vi "Current_and_Spectrum_View.vi"() -> ()   [LabVIEW 2009]
doc: "I. Description:\nThis example demonstrates how to perform an analog software triggered acquisition. The example allows the user to specify the triggering condition and the number of pre-trigger samples to acquire.\n \nII. Instructions for Running:\n1. Select the physical channel to correspond to where your signal is input on the DAQ device.\n2. Enter the minimum and maximum voltage ranges.\nNote: For better accuracy try to match the Input Ranges to the expected voltage level of the measured signal.\n3. Specify the rate of the sample clock. \n4. Specify the number of samples to read per iteration of the continuous input operation. These samples will then be monitored for the trigger condition. The trigger condition is determined by the parameters explained below.\n5. Specify the index of the channel that will be monitored for the requested condition. The first channel in the scan list will have an index equals to 0. It's possible to verify the name of the selected channel once the VI is run, after setting the Channel Index value.\n6. Set the triggering condition to be applied to the channel specified by the Channel Index value. The conditions created for this example are:\n\n- Rising Edge: The trigger condition is met as soon as the monitored signal falls below the Hysteresis window and then crosses past the specified Level.\n- Falling Edge: The trigger condition is met as soon as the monitored signal rises above the Hysteresis window and then crosses past the specified Level.\n- Above Level: The trigger condition is met as soon as the monitored signal is above the specified Level. \n- Below Level: The trigger condition is met as soon as the monitored signal is below the specified Level.\n- When Inside Window: The trigger condition is met as soon as the monitored signal is within the specified window.\n- When Outside Window: The trigger condition is met as soon as the monitored signal is not within the specified window.\n\n7. Set the Level value to be used by the selected condition.\n8. Set the Window Amplitude/ Hysteresis to be used by the Window/Edge conditions\n\n- The upper limit of the conditional window is calculated by adding the Window Amplitude to the condition Level.\n- The lower limit of the conditional window is calculated by subtracting the Window Amplitude from the condition Level.\n- The Hysteresis window for the Rising Edge condition is defined as Level minus the Hysteresis value. \n- The Hysteresis window for the Falling Edge condition is defined as Level plus the Hysteresis value.\n\n8. Set the number of pre-trigger samples if desired.\n\nIII. Block Diagram Steps:\n1. Create an analog input voltage channel.\n2. Find out how many channels are being used in this operation.\n3. Define the Sample Clock Rate. Additionally, define the sample mode to be continuous.\n4. Show the Channel Name of the Condition Channel.\n5. Initialize the data arrays to be used for holding successive iterations of data. This pre-allocation of memory improves the performance of the application. Refer to the VI documentation for more information.\n\nNOTE: The number of samples that meet the triggering condition is not fixed; it depends on the value of the monitored signal. This means that the number of samples to be returned by Analog Trigger Through Software (Scaled).VI may vary from one iteration to the next. In order to avoid dynamically allocating memory while filtering the data (a process that creates), this example pre-allocates arrays for the data before the acquisition starts. The arrays are initialized to the maximum number of elements expected per iteration.\n\n6. Call the Start VI to start the acquisition.\n7. Read the scaled analog input data.\nNote: The Shift Registers attached to the While Loop are used to keep track of triggering status and previous data samples (needed for pre-triggered acquisitions). \n8. Use the Analog Trigger Through Software (Scaled).VI specifically created for this example to detect the requested trigger condition through software.\n9. Show the acquired data if the trigger condition is met.\n10. Stop the loop if the trigger condition is met, an error occurs or the Stop button is pressed. \n11. Call the Clear Task VI to clear the Task.\n12. Use the popup dialog box to display an error or warning if any.\n\nIV. I/O Connections Overview:\nMake sure your signal input terminal matches the Physical Channel I/O control. For further connection information, refer to your hardware reference manual."
uses:
  <vilib>/Utility/error.llb/DialogType.ctl
  <vilib>/DAQmx/configure/timing.llb/DAQmx Timing (Sample Clock).vi
  <vilib>/DAQmx/create/channels.llb/DAQmx Create Channel (AI-Voltage-Basic).vi
  <vilib>/DAQmx/read.llb/DAQmx Read (Analog 2D DBL NChan NSamp).vi
  <vilib>/express/express analysis/Spectral/XNode/ExpressSpectralMeasurementsBlockNode.xnode
  <vilib>/express/express analysis/Spectral/Block/exnSpectralBlock spectral measurements power poly.vi
  <vilib>/express/express analysis/Spectral/Block/exnSpectralBlock spectral measurements power DDT.vi
panel:
  out "x/y":dbl[](array[numeric])
  out "Waveform Graph 2":dynamicdata(graph)
  out "# Pretrigger Samples\nAcquired":i32
  out "Waveform Graph":dbl[][](graph)
  out "Pre-Trigger Error Indicator":bool caption="Error Indicator\n(Indicates if trigger occurs before\npre-trigger samples were acquired)"
  in  "Pretrigger Samples":i32
  in  "Window Amplitude":dbl=0.5 caption="Window Amplitude\n/Hysteresis" step=0.10000000149011612 format="%.2p"
  out "Channel Name":string
  in  "Condition":T1(ring)=enum."Above Level"
  in  "Channel Index":i32
  in  "Level":dbl=-11.0 step=0.10000000149011612 format="%.2p"
  in  "Samples to Read":i32=40000 caption="Samples to Read per Iteration"
  in  "Maximum Value":dbl=10.0 format="%.2p"
  in  "Minimum Value":dbl=-10.0 format="%.2p"
  in  "Physical Channel":tag="Dev1/ai0"
  in  "Rate":dbl=10000.0 caption="Sample Rate (Hz)" format="%0.2f"
  in  "Stop":bool caption="stop"
  # "For instructions, select Help>>Show Context Help"
  # "Channel Parameters"
  # "Timing Parameters"
  # "Triggering Parameters"
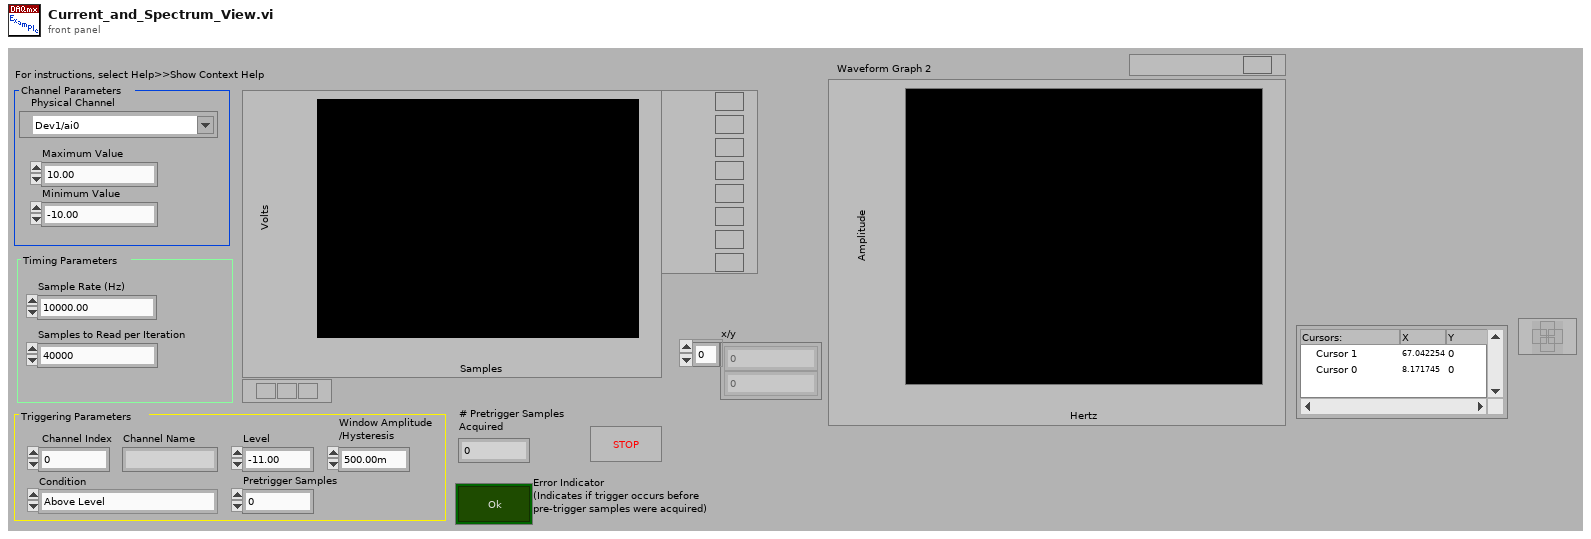
[diagram p1: front panel]
types:
  T1 = enum16{"Rising Edge", "Falling Edge", "Above Level", "Below Level", "When Inside Window", "When Outside Window"}
  T2 = typedef "DialogType.ctl" = u16
  T3 = cluster{"averaging mode":u16, "weighting mode":u16, "number of averages":u32}
  T4 = cluster{"dB On (F)":bool, "unwrap phase (F)":bool, "convert to degree (F)":bool}
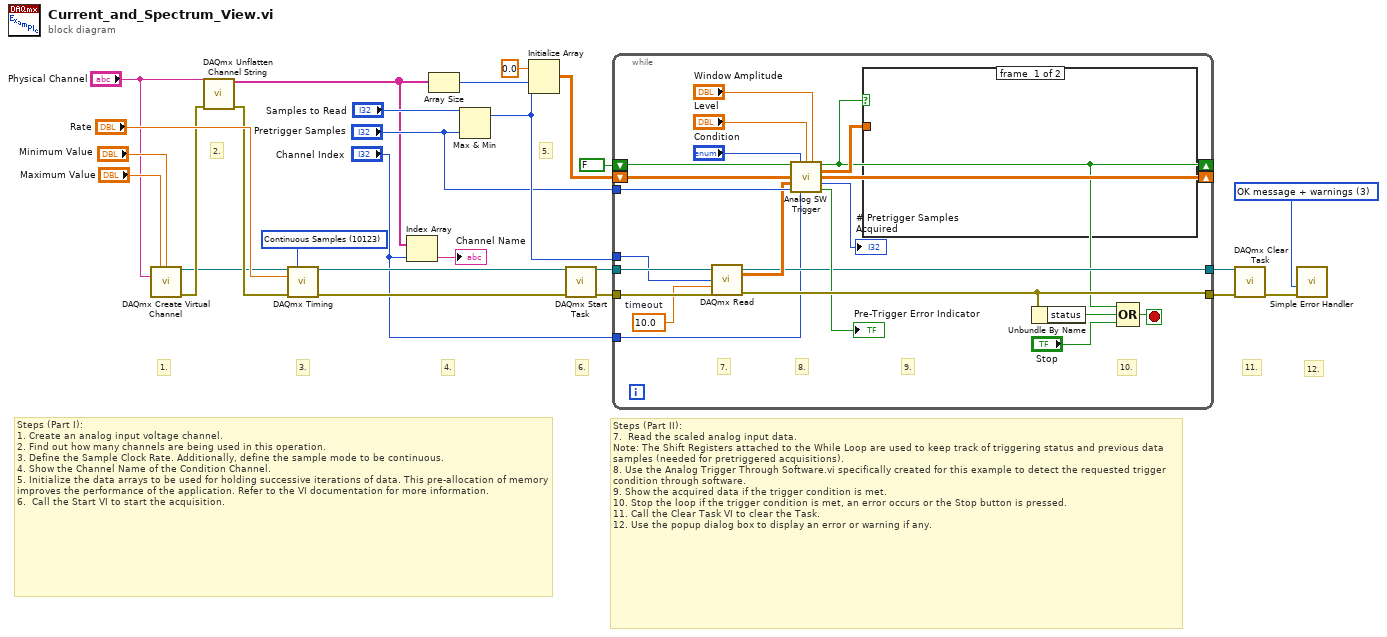
[diagram p0: block diagram]
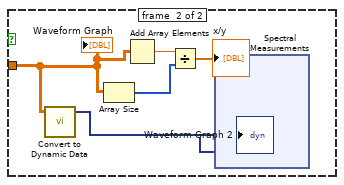
[diagram p2: hidden frame]
diagram:
  w20 = T2 3 items=["no dialog", "OK message", "continue or stop message", "OK message + warnings", "continue/stop + warnings"] ("type of dialog (OK msg:1)")
  w21 = 10123 items=["Finite Samples"=10178, "Continuous Samples"=10123] ("sample mode")
  # "5."
  # "3."
  # "Steps (Part II): \n7.  Read the scaled analog input data.\nNote: The Shift Registers attached to the While Loop are used to keep track of triggering status and previous data samples (needed for pretriggered acquisitions). \n8. Use the Analog Trigger Through Software.vi specifically created for this example to detect the requested trigger condition through software.\n9. Show the acquired data if the trigger condition is met.\n10. Stop the loop if the trigger condition is met, an error occurs or the Stop button is pressed. \n11. Call the Clear Task VI to clear the Task.\n12. Use the popup dialog box to display an error or warning if any."
  # "4."
  # "12."
  # "Steps (Part I): \n1. Create an analog input voltage channel.\n2. Find out how many channels are being used in this operation.\n3. Define the Sample Clock Rate. Additionally, define the sample mode to be continuous.\n4. Show the Channel Name of the Condition Channel.\n5. Initialize the data arrays to be used for holding successive iterations of data. This pre-allocation of memory improves the performance of the application. Refer to the VI documentation for more information.\n6.  Call the Start VI to start the acquisition."
  # "11."
  # "6."
  # "2."
  # "1."
  n1 = call-poly <vilib>:"DAQmx Create Virtual Channel.vi"("maximum value"="Maximum Value", "minimum value"="Minimum Value", "physical channels"="Physical Channel") -> ("task out"=w9:refnum<k21>, "error out"=w14:errorcluster)  [unwired: 11 in]
  n2 = call <vilib>:"DAQmx Unflatten Channel String.vi"("names in"="Physical Channel", "error in"=w14) -> ("names out"=w8:string[], "error out"=w13:errorcluster)  [unwired: 12 in]
  n3 = call-poly <vilib>:"DAQmx Timing.vi"("task/channels in"=w9, "sample mode"=w21, "rate"="Rate", "error in"=w13) -> ("task out"=w5:refnum<k21>, "error out"=w6:errorcluster)  [unwired: 10 in]
  n4 = Index Array(array=w8, index="Channel Index") -> (element=→"Channel Name":string)
  n5 = Array Size(array=w8) -> (size(s)=w2:i32)
  n6 = Max & Min(x="Samples to Read", y="Pretrigger Samples") -> (max(x,y)=w11:i32)  [unwired: 1 out]
  n7 = Initialize Array(0.0, w2, w11) -> (w15:dbl[][])
  n8 = call <vilib>:"DAQmx Start Task.vi"("task/channels in"=w5, "error in"=w6) -> ("task out"=w22:refnum<k21>, "error out"=w24:errorcluster)  [unwired: 12 in]
  n9 = while {
    tunnel: w24 -> [w48]
    tunnel: [w47] -> w17
    tunnel: w22 -> [w46]
    tunnel: [w29] -> w18
    tunnel: w11 -> [w44]
    shift-right: [w27] -> _
    shift-left: FALSE ("stop") -> [w43]
    shift-right: [w32] -> _
    shift-left: w15 -> [w33]
    tunnel: "Pretrigger Samples" -> [w36]
    tunnel: "Channel Index" -> [w28]
    stop <- w38 stop-if-true
    w45 = 10.0  # timeout
    # "10."
    # "9."
    # "7."
    # "8."
    n10 = call-poly <vilib>:"DAQmx Read.vi"("task/channels in"=w46, "number of samples per channel"=w44, "timeout"=w45, "error in"=w48) -> ("task out"=w29:refnum<k21>, "data"=w34:dbl[][], "error out"=w47:errorcluster)  [unwired: 9 in]
    n11 = call "Analog SW Trigger.vi"("Triggered?"=w43, "Condition"="Condition", "Level"="Level", "Window Amplitude"="Window Amplitude", "Initialized Data Array"=w33, "Input Raw Data"=w34, "Pretrigger Samples"=w36, "Index of Condition Channel"=w28) -> ("Trigger Out"=w27:bool, "Output Data (Scaled)"=w31:dbl[][], "Raw Data Out"=w32:dbl[][], "# Pretrigger Samples"=→"# Pretrigger Samples\nAcquired":i32, "Pre-Trigger Error"=→"Pre-Trigger Error Indicator":bool)  [unwired: 3 in]
    n12 = case shown="True" w27 {
      tunnel: w31 -> [_ w52]
      frame #0 {
      }
      frame #1 {
        n13 = call "Convert to Dynamic Data"("2D Array"=w52) -> ("Dynamic Data Type"=w54:dynamicdata)  [unwired: 3 in]
        n14 = Array Size(array=w52) -> (size(s)=w50:i32[])
        n15 = Add Array Elements(numeric array=w52) -> (sum=w51:dbl)
        n16 = Divide(x=w51, y=w50) -> (x/y=→"x/y":dbl[])
        n17 = xnode "Spectral Measurements"("Signals"=w54) -> ("Power Spectrum"=→"Waveform Graph 2":dynamicdata)  [unwired: 1 in, 1 out]
        "Waveform Graph" <- w52
      }
    }
    n18 = Unbundle By Name(w47) -> ("status"=w39:bool)
    n19 = Compound Arithmetic op=OR(w27, w39, "Stop") -> (w38:bool)
  }
  n20 = call <vilib>:"DAQmx Clear Task.vi"("task in"=w18, "error in"=w17) -> ("error out"=w23:errorcluster)  [unwired: 13 in]
  n21 = call <vilib>:"Simple Error Handler.vi"("type of dialog (OK msg:1)"=w20, "error in (no error)"=w23) -> ()  [unwired: 3 in, 5 out]
